vi "Set DS345 wave.vi"(5 "Amplitude (0.01 Vpp)":dbl, 6 "Waveform Function (0: Sine)":u16(ring)=3 items=["Sine", "Square", "Triangle", "Ramp", "Noise"], 7 "Frequency (1000 Hz)":dbl=50.0, 8 "error in (no error)":errorcluster, 11 "VISA resource name":refnum<visa-resource-name>="GPIB0::19::INSTR") -> (0 "error out":errorcluster)   [LabVIEW 2021]
uses:
  <instrlib>/Stanford Research DS345/Stanford Research DS345.lvlib
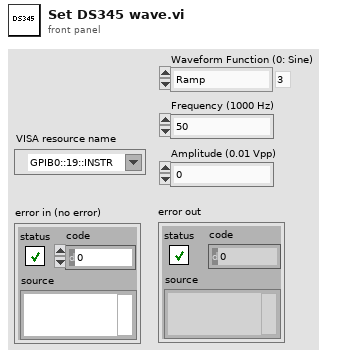
[diagram p1: front panel]
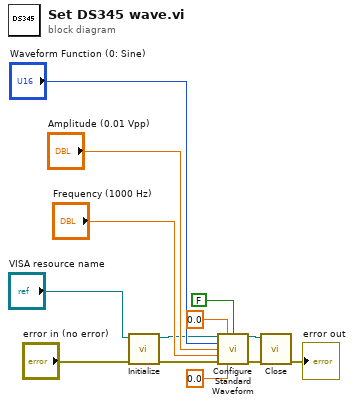
[diagram p0: block diagram]
diagram:
  n1 = call <instrlib>:"Initialize.vi"("error in (no error)"="error in (no error)", "VISA resource name"="VISA resource name") -> ("error out"=w5:errorcluster, "VISA resource name out"=w4:refnum<visa-resource-name>)  [unwired: 8 in]
  n2 = call <instrlib>:"Configure Standard Waveform.vi"("VISA resource name"=w4, "Phase (0.0°)"=0.0, "Enable Output Inversion (F: Disable)"=FALSE, "Waveform Function (0: Sine)"="Waveform Function (0: Sine)", "Amplitude (0.01 Vpp)"="Amplitude (0.01 Vpp)", "Frequency (1000 Hz)"="Frequency (1000 Hz)", "error in (no error)"=w5, "DC Offset (0.00 V)"=0.0) -> ("VISA resource name out"=w1:refnum<visa-resource-name>, "error out"=w3:errorcluster)  [unwired: 6 in]
  n3 = call <instrlib>:"Close.vi"("error in (no error)"=w3, "VISA resource name"=w1) -> ("error out"=→"error out":errorcluster)  [unwired: 9 in]
